vi "ADI_IMU_ADIS16448_CRC.vi"(7 "Look-Up Table Method?":bool, 10 "Byte Array (MSB-First)":u8[](array[numeric])) -> (2 "CRC16-ADIS":u16)   [LabVIEW 2017, in "ADIS16448_IMU.lvlib"]
uses:
  ADIS16448_IMU.lvlib
panel:
  out "Generated \nCRC-16 Lookup Table":u16[](array[numeric]) format="%04x"
  # "This vi calculates a CRC16 check on data generated from an \nADIS16448 IMU when using burst mode (MSC_CTRL[4] = 1). \nThis implementation is a variant of the CCITT X.25 spec.\n\nJuan Chong - December 2017"
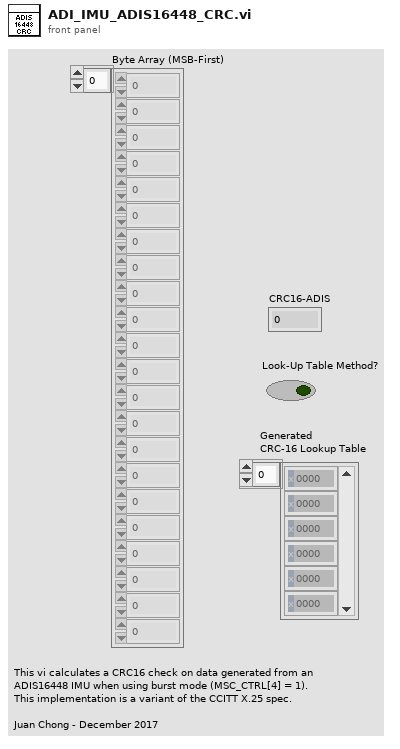
[diagram p1: front panel]
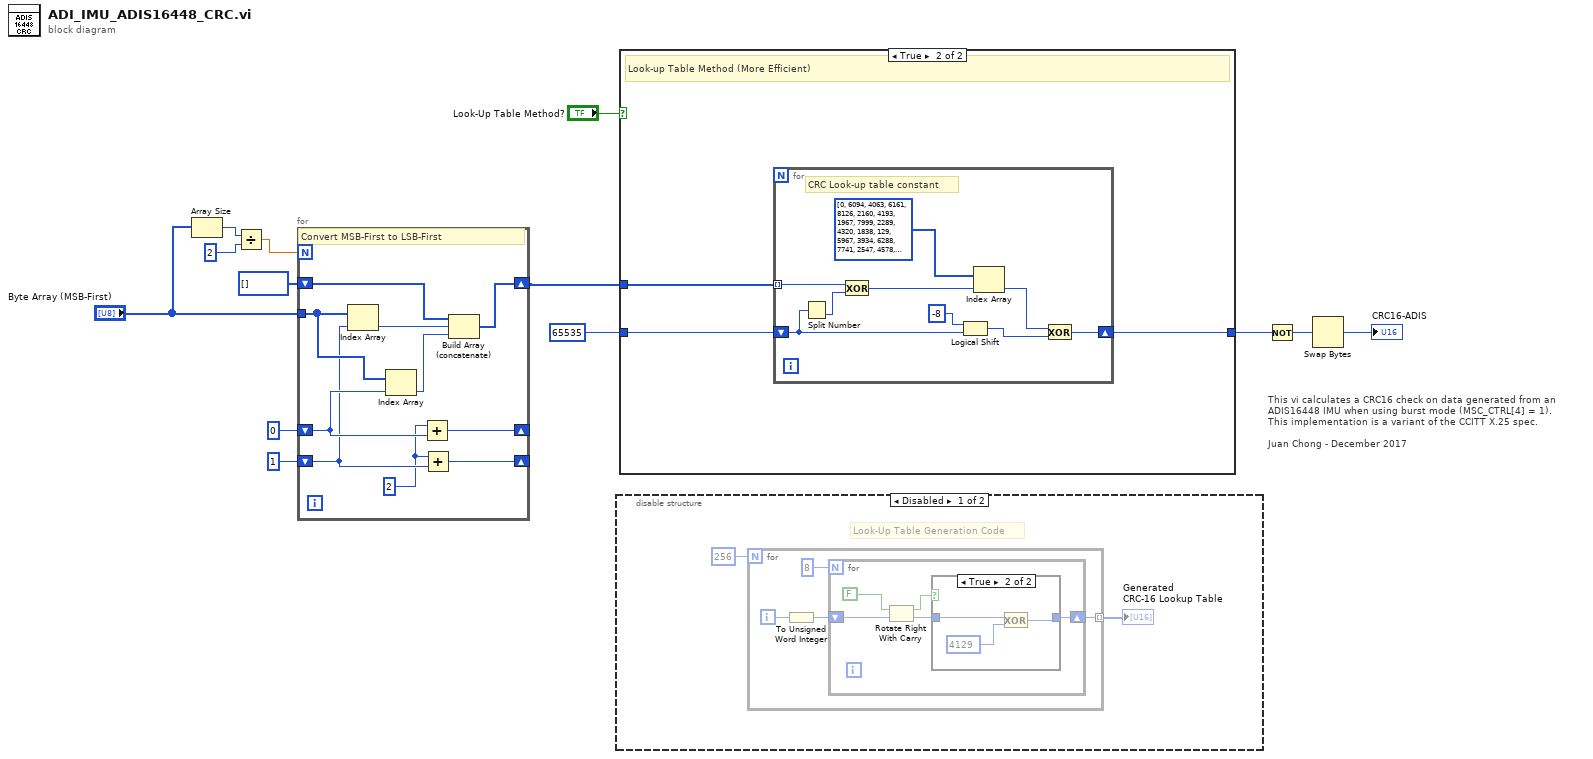
[diagram p0: block diagram]
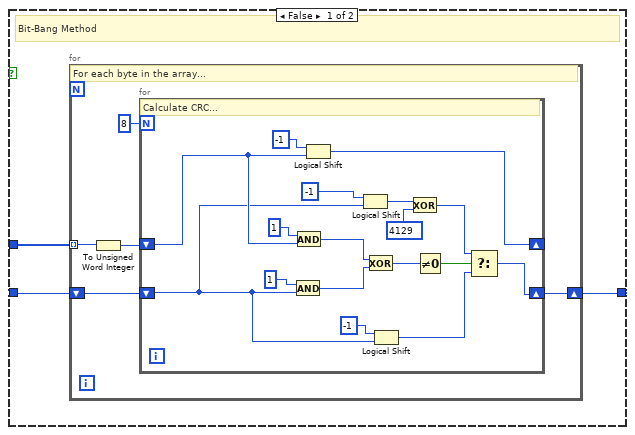
[diagram p4: hidden frame]
diagram:
  # "This vi calculates a CRC16 check on data generated from an \nADIS16448 IMU when using burst mode (MSC_CTRL[4] = 1). \nThis implementation is a variant of the CCITT X.25 spec.\n\nJuan Chong - December 2017"
  n1 = Array Size(array="Byte Array (MSB-First)") -> (size(s)=w4:i32)
  n2 = Divide(x=w4, y=2) -> (x/y=w3:dbl)
  n3 = for {
    N: w3 -> [_]
    tunnel: "Byte Array (MSB-First)" -> [w23]
    shift-right: [w20] -> _
    shift-left: 0 -> [w22]
    shift-right: [w21] -> _
    shift-left: 1 -> [w19]
    shift-right: [w15] -> w2
    shift-left: u8[] [] -> [w14]
    w18 = 2 ("x")
    # "Convert MSB-First to LSB-First"
    n4 = Index Array(array=w23, index=w19) -> (element=w17:u8)
    n5 = Index Array(array=w23, index=w22) -> (element=w16:u8)
    n6 = Add(x=w18, y=w22) -> (x+y=w20:i32)
    n7 = Add(x=w18, y=w19) -> (x+y=w21:i32)
    n8 = Build Array (concatenate)(w14, w17, w16) -> (w15:u8[])
  }
  n9 = disable-structure shown="Disabled" {
    frame Disabled {
      # "Look-Up Table Generation Code"
      n10 = for {
        N: 256 -> [_]
        tunnel: [w28] -> w24 mode=indexing
        i -> [w27]
        n11 = To Unsigned Word Integer(number=w27) -> (unsigned 16bit integer=w26:u16)
        n12 = for {
          N: 8 -> [_]
          shift-right: [w31] -> w28
          shift-left: w26 -> [w30]
          n13 = Rotate Right With Carry(2:w30, 3:FALSE) -> (0:w32:u16, 1:w33:bool)
          n14 = case shown="True" w33 {
            tunnel: w32 -> [w35 w38]
            tunnel: [w35 w36] -> w31
            frame False {
            }
            frame True {
              n15 = Exclusive Or(1:u16 4129, 2:w38) -> (0:w36:u16)
            }
          }
        }
      }
      "Generated \nCRC-16 Lookup Table" <- w24
    }
    frame Enabled {
    }
  }
  n16 = case shown="True" "Look-Up Table Method?" {
    tunnel: w2 -> [w41 w66]
    tunnel: [w40 w65] -> w13
    tunnel: u16 65535 -> [w39 w64]
    frame False {
      # "Bit-Bang Method"
      n17 = for {
        tunnel: w41 -> [w43] mode=indexing
        shift-right: [w45] -> w40
        shift-left: w39 -> [w46]
        # "For each byte in the array..."
        n18 = To Unsigned Word Integer(number=w43) -> (unsigned 16bit integer=w42:u16)
        n19 = for {
          N: 8 -> [_]
          shift-right: [w53] -> w45
          shift-left: w46 -> [w47]
          shift-right: [w49] -> _
          shift-left: w42 -> [w48]
          # "Calculate CRC..."
          n20 = And(x=u16 1, y=w47) -> (x .and. y?=w62:u16)
          n21 = And(x=u16 1, y=w48) -> (x .and. y?=w51:u16)
          n22 = Logical Shift(y=i16 -1, x=w48) -> (x << y=w49:u16)
          n23 = Logical Shift(y=i16 -1, x=w47) -> (x << y=w58:u16)
          n24 = Exclusive Or(1:w62, 2:w51) -> (0:w61:u16)
          n25 = Logical Shift(y=i16 -1, x=w47) -> (x << y=w54:u16)
          n26 = Exclusive Or(1:u16 4129, 2:w58) -> (0:w56:u16)
          n27 = Not Equal To 0?(x=w61) -> (x != 0?=w60:bool)
          n28 = Select(t=w56, s=w60, f=w54) -> (s? t:f=w53:u16)
        }
      }
    }
    frame True {
      # "Look-up Table Method (More Efficient)"
      n29 = for {
        tunnel: w66 -> [w69] mode=indexing
        shift-right: [w73] -> w65
        shift-left: w64 -> [w71]
        # "CRC Look-up table constant"
        n30 = Split Number(x=w71) -> (lo(x)=w70:u8)  [unwired: 1 out]
        n31 = Exclusive Or(1:w70, 2:w69) -> (0:w68:u8)
        n32 = Logical Shift(y=i8 -8, x=w71) -> (x << y=w74:u16)
        n33 = Index Array(array=u16[] [0, 6094, 4063, 6161, 8126, 2160, 4193, 1967, 7999, 2289, 4320, 1838, 129, 5967, 3934, 6288, 7741, 2547, 4578, 1580, 387, 5709, 3676, 6546, 258, 5836, 3805, 6419, 7868, 2418, 4451, 1709, 7225, 3063, 5094, 1064, 903, 5193, 3160, 7062, 774, 5320, 3289, 6935, 7352, 2934, 4967, 1193, 516, 5578, 3547, 6677, 7610, 2676, 4709, 1451, 7483, 2805, 4836, 1322, 645, 5451, 3418, 6804, 6193, 4095, 6126, 32, 1935, 4161, 2128, 8094, 1806, 4288, 2257, 7967, 6320, 3966, 5999, 161, 1548, 4546, 2515, 7709, 6578, 3708, 5741, 419, 6451, 3837, 5868, 290, 1677, 4419, 2386, 7836, 1032, 5062, 3031, 7193, 7094, 3192, 5225, 935, 6967, 3321, 5352, 806, 1161, 4935, 2902, 7320, 6709, 3579, 5610, 548, 1419, 4677, 2644, 7578, 1290, 4804, 2773, 7451, 6836, 3450, 5483, 677, 4129, 2031, 8190, 2096, 3999, 6225, 64, 6030, 3870, 6352, 193, 5903, 4256, 1902, 8063, 2225, 3612, 6610, 451, 5645, 4514, 1644, 7805, 2483, 4387, 1773, 7932, 2354, 3741, 6483, 322, 5772, 3096, 7126, 967, 5129, 5030, 1128, 7289, 2999, 4903, 1257, 7416, 2870, 3225, 6999, 838, 5256, 4645, 1515, 7674, 2612, 3483, 6741, 580, 5514, 3354, 6868, 709, 5387, 4772, 1386, 7547, 2741, 2064, 8158, 1999, 4097, 6062, 96, 6257, 4031, 5935, 225, 6384, 3902, 2193, 8031, 1870, 4224, 5677, 483, 6642, 3644, 2451, 7773, 1612, 4482, 2322, 7900, 1741, 4355, 5804, 354, 6515, 3773, 5161, 999, 7158, 3128, 2967, 7257, 1096, 4998, 2838, 7384, 1225, 4871, 5288, 870, 7031, 3257, 2580, 7642, 1483, 4613, 5546, 612, 6773, 3515, 5419, 741, 6900, 3386, 2709, 7515, 1354, 4740] ("CRC-16 Lookup Table 2"), index=w68) -> (element=w72:u16)
        n34 = Exclusive Or(1:w74, 2:w72) -> (0:w73:u16)
      }
    }
  }
  n35 = Not(x=w13) -> (.not. x?=w12:u16)
  n36 = Swap Bytes(anything=w12) -> (byte swapped=→"CRC16-ADIS":u16)
